vi "Change Setting.vi"(8 "error in (no error)":errorcluster, 10 "Change setting mode":T1=enum."Next", 11 "NI DAQmx in":refnum<class "NI DAQmx.lvclass">) -> (0 "error out":errorcluster, 1 "Changes":cluster{"Name":string, "Value":string}[](array[cluster]), 2 "Last setting":bool, 3 "NI DAQmx out":refnum<class "NI DAQmx.lvclass">)   [LabVIEW 2020, in "NI DAQmx.lvclass"]
uses:
  NI DAQmx.lvclass
  C:/Sandbox/RF Bench/Source Code/WiSpry Test Framework/Devices/Device.lvclass
  Controls/Change setting mode enum.ctl
  <vilib>/DAQmx/write.llb/DAQmx Write (Digital Bool 1Line 1Point).vi
  <vilib>/DAQmx/read.llb/DAQmx Read (Digital Bool 1Line 1Point).vi
  <vilib>/DAQmx/miscellaneous.llb/DAQmx Fill In Error Info.vi
  PIC-device/PIC-Device.lvclass
panel:
  out "All ok":bool
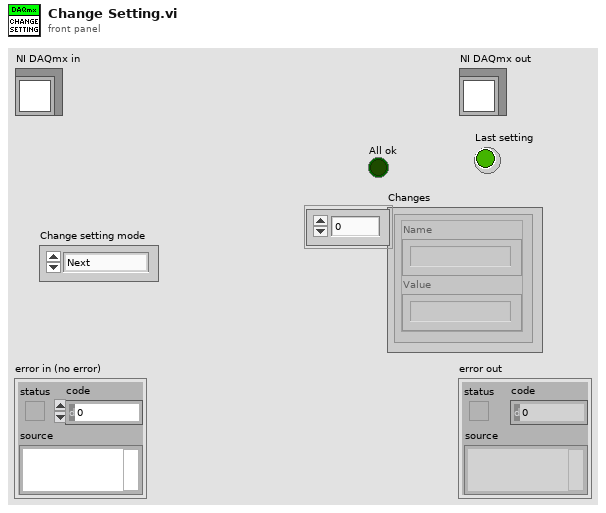
[diagram p1: front panel]
types:
  T1 = typedef "PIC-Device.lvclass/Change setting mode enum.ctl" = enum16{"Init", "Next", "Reset"}
  T2 = cluster{"GPIO Settings":bool[][], "GPIO Values":string[]}
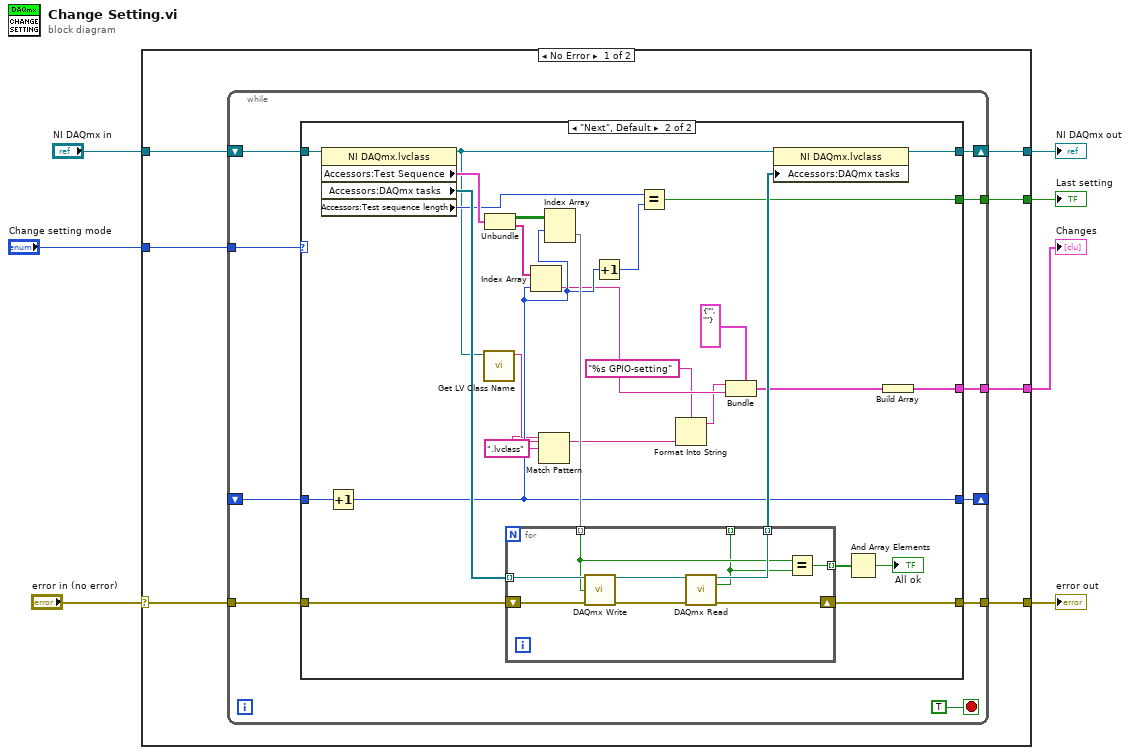
[diagram p0: block diagram]
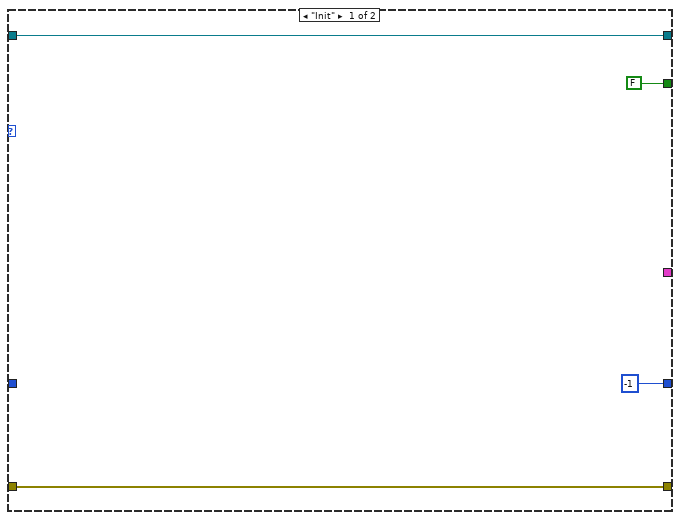
[diagram p2: hidden frame]
diagram:
  n1 = case shown="No Error" "error in (no error)" {
    selector: "error in (no error)" -> [w10 w66]
    tunnel: [w11 w66] -> w6
    tunnel: "NI DAQmx in" -> [w12 w65]
    tunnel: [w9 w65] -> w4
    tunnel: "Change setting mode" -> [w14 _]
    tunnel: [w13 _] -> w2
    tunnel: [w8 _] -> w1
    frame No Error {
      n2 = while {
        tunnel: w14 -> [w24]
        tunnel: [w22] -> w13
        shift-right: [w21] -> _
        shift-left: _ -> [w20]
        tunnel: [w18] -> w11
        tunnel: w10 -> [w17]
        shift-right: [w16] -> w9
        shift-left: w12 -> [w19]
        tunnel: [w15] -> w8
        stop <- TRUE stop-if-true
        n3 = case shown="\"Next\", Default" w24 {
          tunnel: [FALSE w43] -> w22
          tunnel: [-1 w42] -> w21
          tunnel: w20 -> [_ w46]
          tunnel: w19 -> [w25 w55]
          tunnel: [w26 w48] -> w18
          tunnel: w17 -> [w26 w47]
          tunnel: [w25 w45] -> w16
          tunnel: [_ w34] -> w15
          frame "Init" {
          }
          frame "Next", Default {
            n4 = property class="NI DAQmx.lvclass"(reference=w55) -> (reference out=w38:refnum<class "NI DAQmx.lvclass">, "Accessors:Test Sequence"=w54:T2, "Accessors:DAQmx tasks"=w53:refnum<k21>[], "Accessors:Test sequence length"=w44:i32)  [unwired: 1 in, 1 out]
            n5 = Increment(x=w46) -> (x+1=w42:i32)
            n6 = call <vilib>:"Get LV Class Name.vi"("object"=w38) -> ("class name"=w33:string)  [unwired: 9 in, 1 out]
            n7 = Unbundle(w54) -> ("GPIO Settings"=w51:bool[][], "GPIO Values"=w49:string[])
            n8 = Index Array(array=w49, index=w42) -> (element=w39:string)
            n9 = Match Pattern(string=w33, regular expression=".lvclass") -> (before substring=w31:string)  [unwired: 1 in, 3 out]
            n10 = Index Array(array=w51, index (row)=w42) -> (element=w50:bool[])  [unwired: 1 in]
            n11 = for {
              tunnel: w53 -> [w62] mode=indexing
              tunnel: [w61] -> w52 mode=indexing
              tunnel: w50 -> [w58] mode=indexing
              tunnel: [w57] -> _ mode=indexing
              shift-right: [w60] -> w48
              shift-left: w47 -> [w59]
              tunnel: [w56] -> w30 mode=indexing
              n12 = call-poly <vilib>:"DAQmx Write.vi"("task/channels in"=w62, "data"=w58, "error in"=w59) -> ("task out"=w64:refnum<k21>, "error out"=w63:errorcluster)  [unwired: 10 in, 1 out]
              n13 = call-poly <vilib>:"DAQmx Read.vi"("task/channels in"=w64, "error in"=w63) -> ("task out"=w61:refnum<k21>, "data"=w57:bool, "error out"=w60:errorcluster)  [unwired: 11 in]
              n14 = Equal?(x=w58, y=w57) -> (x = y?=w56:bool)
            }
            n15 = Increment(x=w42) -> (x+1=w41:i32)
            n16 = Equal?(x=w44, y=w41) -> (x = y?=w43:bool)
            n17 = Format Into String(format string="%s GPIO-setting" ("Name"), w31) -> (resulting string=w36:string)  [unwired: 2 in, 1 out]
            n18 = Bundle(cluster=cluster{"Name":string, "Value":string} {"Name"="", "Value"=""} ("Change"), "Name"=w36, "Value"=w39) -> (w35:cluster{"Name":string, "Value":string})
            n19 = property class="NI DAQmx.lvclass"(reference=w38, "Accessors:DAQmx tasks"=w52) -> (reference out=w45:refnum<class "NI DAQmx.lvclass">)  [unwired: 1 in, 1 out]
            n20 = And Array Elements(Boolean array=w30) -> (logical AND=→"All ok":bool)
            n21 = Build Array(w35) -> (w34:cluster{"Name":string, "Value":string}[])
          }
        }
      }
    }
    frame Error {
    }
  }
  "error out" <- w6
  "NI DAQmx out" <- w4
  "Changes" <- w1
  "Last setting" <- w2
